vi "Clear Warnings.vi"(1 "error in (no error)":errorcluster) -> (0 "error out":errorcluster)   [LabVIEW 2011]
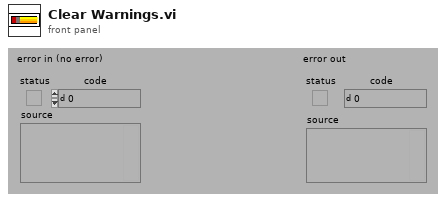
[diagram p1: front panel]
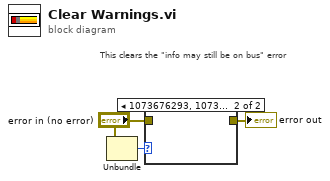
[diagram p0: block diagram]
diagram:
  # "This clears the \"info may still be on bus\" error"
  n1 = Unbundle("error in (no error)") -> ("code"=w3:i32)  [unwired: 2 out]
  n2 = case shown="1073676293, 1073676294" w3 {
    tunnel: "error in (no error)" -> [w4 _]
    tunnel: [w4 _] -> w1
    frame Default {
    }
    frame 1073676293, 1073676294 {
    }
  }
  "error out" <- w1
